vi "FuncImg-Get number of points in single ROI trial.vi"(8 "Error in":errorcluster, 11 "Single ROI data files reorderedin ascending file-name order":path[](array[path])) -> (0 "Error out":errorcluster, 2 "Number of data points in single POI (all trials)":i32)   [LabVIEW 2013]
uses:
  Program Files (x86)/National Instruments/LabVIEW 2013/user.lib/My Palettes.lib/Files & paths/Spreadsheet/Read From Spreadsheet File (I64)-Mod.vi
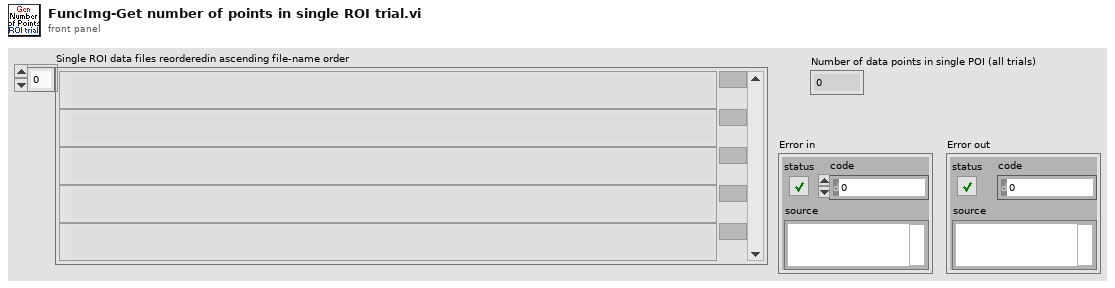
[diagram p1: front panel]
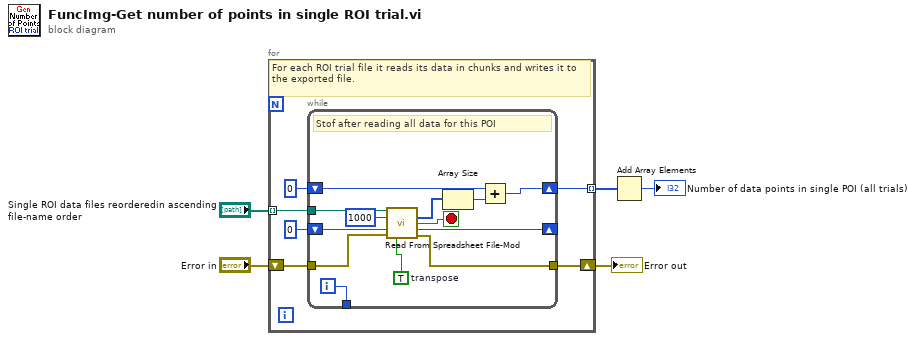
[diagram p0: block diagram]
diagram:
  n1 = for {
    tunnel: "Single ROI data files reorderedin ascending file-name order" -> [w11] mode=indexing
    tunnel: [w10] -> w4 mode=indexing
    shift-right: [w7] -> w1
    shift-left: "Error in" -> [w6]
    # "For each ROI trial file it reads its data in chunks and writes it to the exported file."
    n2 = while {
      tunnel: w11 -> [w22]
      shift-right: [w17] -> w10
      shift-left: 0 ("start of read offset (chars.:0)") -> [w19]
      shift-right: [w16] -> _
      shift-left: 0 ("start of read offset (chars.:0)") -> [w21]
      tunnel: [w15] -> _
      tunnel: [w14] -> w7
      tunnel: w6 -> [w12]
      i -> [w15]
      stop <- w13 stop-if-true
      w24 = TRUE  # transpose
      # "Stof after reading all data for this POI"
      n3 = call-poly "Read From Spreadsheet File-Mod.vi"("file path (dialog if empty)"=w22, "number of rows (all:-1)"=1000, "start of read offset (chars.:0)"=w21, "error in"=w12, "transpose (no:F)"=w24) -> ("first row"=w23:i64[], "EOF?"=w13:bool, "mark after read (chars.)"=w16:i32, "error out"=w14:errorcluster)  [unwired: 5 in, 2 out]
      n4 = Array Size(array=w23) -> (size(s)=w20:i32)
      n5 = Add(x=w19, y=w20) -> (x+y=w17:i32)
    }
  }
  "Error out" <- w1
  n6 = Add Array Elements(numeric array=w4) -> (sum=→"Number of data points in single POI (all trials)":i32)
